vi "Color Boxes.vi"() -> ()   [LabVIEW 2017]
panel:
  out "Our Switch (R)":u32(colorbox)
  out "Our Switch (L)":u32(colorbox)
  out "Other Switch (R)":u32(colorbox)
  out "Other Switch (L)":u32(colorbox)
  out "Scale (L)":u32(colorbox)
  in  "Colour":enum16{"Blue", "Red"}(ring)
  in  "Game Data":string
  out "Scale (R)":u32(colorbox)
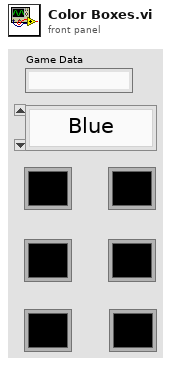
[diagram p1: front panel]
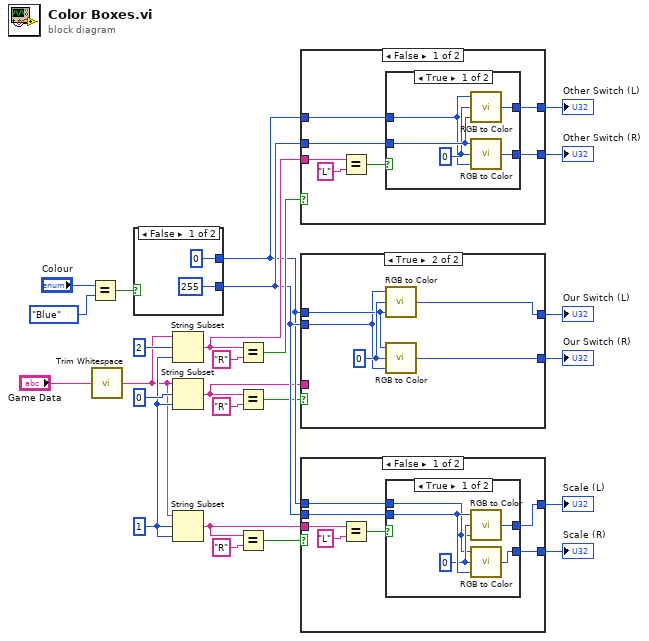
[diagram p0: block diagram]
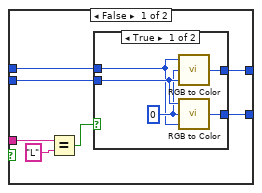
[diagram p2: hidden frame]
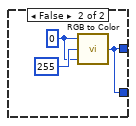
[diagram p3: hidden frame]
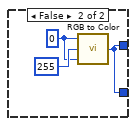
[diagram p4: hidden frame]
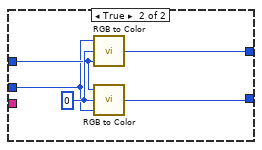
[diagram p5: hidden frame]
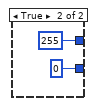
[diagram p6: hidden frame]
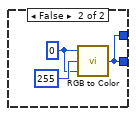
[diagram p7: hidden frame]
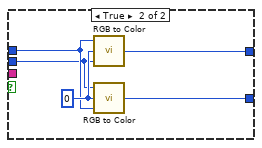
[diagram p8: hidden frame]
diagram:
  w19 = 1 ("length (rest)")
  n1 = Equal?(x="Colour", y=enum16{"Blue", "Red"}."Blue") -> (x = y?=w14:bool)
  n2 = call <vilib>:"Trim Whitespace.vi"("string"="Game Data") -> ("trimmed string"=w17:string)  [unwired: 1 in]
  n3 = case shown="False" w14 {
    tunnel: [u8 0 ("R") u8 255 ("R")] -> w7
    tunnel: [u8 255 ("R") u8 0 ("R")] -> w8
    frame False {
    }
    frame True {
    }
  }
  n4 = String Subset(string=w17, offset (0)=2, length (rest)=w19) -> (substring=w12:string)
  n5 = String Subset(string=w17, offset (0)=0, length (rest)=w19) -> (substring=w6:string)
  n6 = String Subset(string=w17, offset (0)=w19, length (rest)=w19) -> (substring=w21:string)
  n7 = Equal?(x=w12, y="R") -> (x = y?=w11:bool)
  n8 = Equal?(x=w6, y="R") -> (x = y?=w5:bool)
  n9 = Equal?(x=w21, y="R") -> (x = y?=w23:bool)
  n10 = case shown="False" w11 {
    tunnel: [w33 w49] -> w10
    tunnel: w12 -> [w35 _]
    tunnel: w8 -> [w32 w45]
    tunnel: w7 -> [w31 w46]
    tunnel: [w30 w47] -> w9
    frame False {
      n11 = Equal?(x=w35, y="L") -> (x = y?=w36:bool)
      n12 = case shown="True" w36 {
        tunnel: [w38 w42] -> w33
        tunnel: w32 -> [w41 _]
        tunnel: w31 -> [w39 _]
        tunnel: [w37 w42] -> w30
        frame True {
          w40 = u8 0 ("B")
          n13 = call <vilib>:"RGB to Color.vi"("B"=w41, "G"=w40, "R"=w39) -> ("Color"=w38:u32)
          n14 = call <vilib>:"RGB to Color.vi"("B"=w39, "G"=w40, "R"=w41) -> ("Color"=w37:u32)
        }
        frame False {
          w43 = u8 0 ("B")
          n15 = call <vilib>:"RGB to Color.vi"("B"=w43, "G"=u8 255 ("R"), "R"=w43) -> ("Color"=w42:u32)
        }
      }
    }
    frame True {
      w48 = u8 0 ("B")
      n16 = call <vilib>:"RGB to Color.vi"("B"=w46, "G"=w48, "R"=w45) -> ("Color"=w49:u32)
      n17 = call <vilib>:"RGB to Color.vi"("B"=w45, "G"=w48, "R"=w46) -> ("Color"=w47:u32)
    }
  }
  "Other Switch (L)" <- w10
  "Other Switch (R)" <- w9
  n18 = case shown="True" w5 {
    tunnel: [w53 w69] -> w4
    tunnel: w6 -> [w55 _]
    tunnel: w8 -> [w52 w65]
    tunnel: w7 -> [w51 w66]
    tunnel: [w50 w67] -> w3
    frame False {
      n19 = Equal?(x=w55, y="L") -> (x = y?=w56:bool)
      n20 = case shown="True" w56 {
        tunnel: [w58 w62] -> w53
        tunnel: w52 -> [w61 _]
        tunnel: w51 -> [w59 _]
        tunnel: [w57 w62] -> w50
        frame True {
          w60 = u8 0 ("B")
          n21 = call <vilib>:"RGB to Color.vi"("B"=w61, "G"=w60, "R"=w59) -> ("Color"=w58:u32)
          n22 = call <vilib>:"RGB to Color.vi"("B"=w59, "G"=w60, "R"=w61) -> ("Color"=w57:u32)
        }
        frame False {
          w63 = u8 0 ("B")
          n23 = call <vilib>:"RGB to Color.vi"("B"=w63, "G"=u8 255 ("R"), "R"=w63) -> ("Color"=w62:u32)
        }
      }
    }
    frame True {
      w68 = u8 0 ("B")
      n24 = call <vilib>:"RGB to Color.vi"("B"=w66, "G"=w68, "R"=w65) -> ("Color"=w69:u32)
      n25 = call <vilib>:"RGB to Color.vi"("B"=w65, "G"=w68, "R"=w66) -> ("Color"=w67:u32)
    }
  }
  "Our Switch (L)" <- w4
  "Our Switch (R)" <- w3
  n26 = case shown="False" w23 {
    tunnel: [w73 w89] -> w2
    tunnel: w21 -> [w75 _]
    tunnel: w8 -> [w72 w85]
    tunnel: w7 -> [w71 w86]
    tunnel: [w70 w87] -> w13
    frame False {
      n27 = Equal?(x=w75, y="L") -> (x = y?=w76:bool)
      n28 = case shown="True" w76 {
        tunnel: [w78 w82] -> w73
        tunnel: w72 -> [w81 _]
        tunnel: w71 -> [w79 _]
        tunnel: [w77 w82] -> w70
        frame True {
          w80 = u8 0 ("B")
          n29 = call <vilib>:"RGB to Color.vi"("B"=w79, "G"=w80, "R"=w81) -> ("Color"=w77:u32)
          n30 = call <vilib>:"RGB to Color.vi"("B"=w81, "G"=w80, "R"=w79) -> ("Color"=w78:u32)
        }
        frame False {
          w83 = u8 0 ("B")
          n31 = call <vilib>:"RGB to Color.vi"("B"=w83, "G"=u8 255 ("R"), "R"=w83) -> ("Color"=w82:u32)
        }
      }
    }
    frame True {
      w88 = u8 0 ("B")
      n32 = call <vilib>:"RGB to Color.vi"("B"=w85, "G"=w88, "R"=w86) -> ("Color"=w87:u32)
      n33 = call <vilib>:"RGB to Color.vi"("B"=w86, "G"=w88, "R"=w85) -> ("Color"=w89:u32)
    }
  }
  "Scale (R)" <- w2
  "Scale (L)" <- w13
